vi "Write wave DRAM index control.vi"(11 "Current index":i32) -> (1 "Output Valid":bool, 2 "Next index":i32, 3 "Current index":i32)   [LabVIEW 2015]
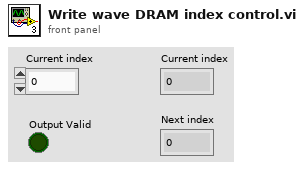
[diagram p1: front panel]
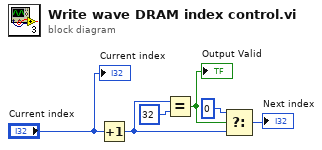
[diagram p0: block diagram]
diagram:
  n1 = Increment(x="Current index") -> (x+1=w5:i32)
  n2 = Equal?(x=w5, y=32) -> (x = y?=w2:bool)
  "Output Valid" <- w2
  n3 = Select(t=0, s=w2, f=w5) -> (s? t:f=→"Next index":i32)
  "Current index" <- "Current index"
